vi "TAT-T-Alarm Display.vi"(11 "T-Alarm":u16[](array[numeric]) format="%b") -> ()   [LabVIEW 2017]
panel:
  in  "stop":bool
  out "Alarm List":string
  # "TORQUE ALARMS"
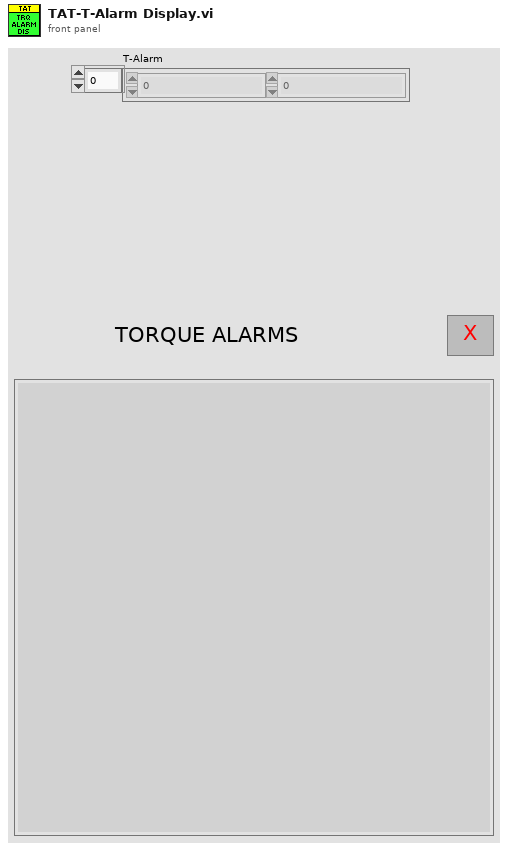
[diagram p1: front panel]
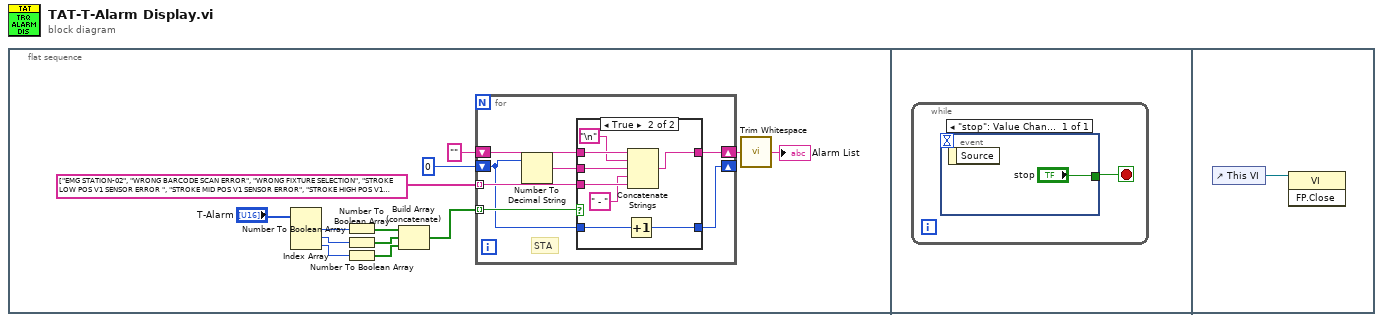
[diagram p0: block diagram]
diagram:
  n1 = flat-sequence {
    frame #0 {
      n2 = Index Array(array="T-Alarm") -> (element #1=w7:u16, element #2=w6:u16, element #3=w5:u16)  [unwired: 3 in]
      n3 = Number To Boolean Array(number=w7) -> (Boolean array=w4:bool[])
      n4 = Number To Boolean Array(number=w6) -> (Boolean array=w3:bool[])
      n5 = Number To Boolean Array(number=w5) -> (Boolean array=w2:bool[])
      n6 = Build Array (concatenate)(w4, w3, w2) -> (w1:bool[])
      n7 = for {
        tunnel: w1 -> [w19] mode=indexing
        tunnel: string[] ["EMG STATION-02", "WRONG BARCODE SCAN ERROR", "WRONG FIXTURE SELECTION", "STROKE LOW POS V1 SENSOR ERROR ", "STROKE MID POS V1 SENSOR ERROR", "STROKE HIGH POS V1 SENSOR ERROR ", "STROKE LOW POS V2 SENSOR ERROR", "STROKE MID POS V2 SENSOR ERROR", "STROKE HIGH POS V2 SENSOR ERROR", "TORQUEING STATION BRACKET SENSOR-01", "", "", "", "", "", "", "TORQUEING STATION BRACKET SENSOR-02", "TORQUEING STATION BRACKET SENSOR-03", "TORQUEING STATION BRACKET SENSOR-04", "TORQUEING STATION BRACKET SENSOR-05", "TORQUEING STATION BRACKET SENSOR-06", "TORQUEING STATION BRACKET SENSOR-07", "TORQUEING STATION BRACKET SENSOR-08", "TORQUEING STATION STUD PRESENT SENSOR ERROR-09", "TORQUEING STATION STUD PRESENT SENSOR ERROR-10", "TORQUEING STATION STUD PRESENT SENSOR ERROR-11", "", "", "", "", "", "", "TORQUEING STATION STUD PRESENT SENSOR ERROR-12", "DOT PUNCH CYLINDER FW REED SW", "TORQUE GUN NOK"] -> [w17] mode=indexing
        shift-right: [w18] -> w11
        shift-left: "" -> [w20]
        shift-right: [w15] -> _
        shift-left: u8 0 -> [w14]
        # "STA"
        n8 = Number To Decimal String(number=w14) -> (decimal integer string=w16:string)  [unwired: 1 in]
        n9 = case shown="True" w19 {
          tunnel: w20 -> [w22 w30]
          tunnel: [w22 w28] -> w18
          tunnel: w17 -> [_ w26]
          tunnel: w16 -> [_ w27]
          tunnel: [w21 w23] -> w15
          tunnel: w14 -> [w21 w24]
          frame False {
          }
          frame True {
            n10 = Increment(x=w24) -> (x+1=w23:u8)
            n11 = Concatenate Strings(w30, "\n", w27, " - ", w26) -> (w28:string)
          }
        }
      }
      n12 = call <vilib>:"Trim Whitespace.vi"("string"=w11) -> ("trimmed string"=→"Alarm List":string)  [unwired: 1 in]
    }
    frame #1 {
      n13 = while {
        stop <- w31 stop-if-true
        n14 = event shown="[0] \"stop\": Value Change" {
          selector: _ -> [_]
          dyn-events: _ -> [_]
          timeout: _ -> [_]
          tunnel: ["stop"] -> w31
          event "stop": Value Change {
            n15 = event-data() -> ()  [unwired: 1 in, 1 out]
          }
        }
      }
    }
    frame #2 {
      n16 = control-ref of="This VI"() -> (w33:refnum<vi>)
      n17 = invoke class="VI" method="FP.Close"(reference=w33) -> ()  [unwired: 2 in, 3 out]
    }
  }
